vi "Serialize - Text.vi"(8 "error in (no error)":errorcluster, 11 "CRDS Data in":refnum<class "CRDS Data.lvclass">) -> (0 "error out":errorcluster, 2 "Serialized Text":string, 3 "CRDS Data out":refnum<class "CRDS Data.lvclass">)   [LabVIEW 2014, in "CRDS Lib.lvlib" / "CRDS Data.lvclass"]
uses:
  CRDS Data.lvclass
  CRDS Data.lvclass/CRDS Data.ctl
  Cell/CRDS Cell Data.lvclass
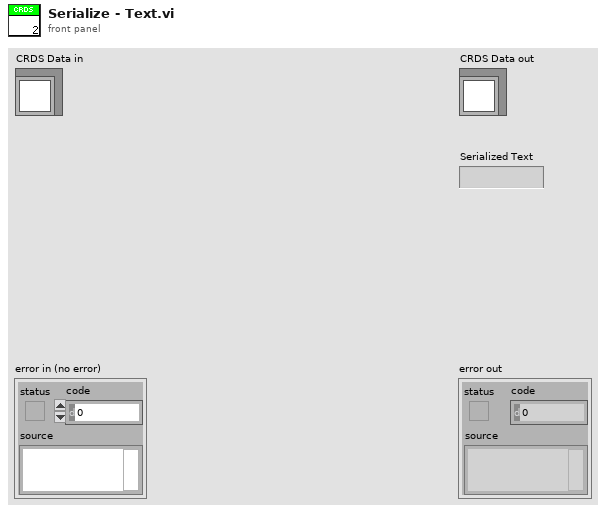
[diagram p1: front panel]
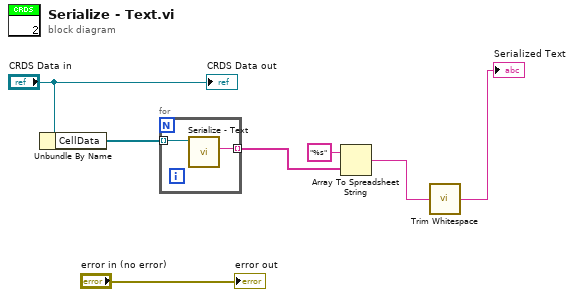
[diagram p0: block diagram]
diagram:
  n1 = Unbundle By Name("CRDS Data in") -> ("CellData"=w5:refnum<class "CRDS Cell Data.lvclass">[])
  n2 = for {
    tunnel: w5 -> [w9] mode=indexing
    tunnel: [w8] -> w4 mode=indexing
    n3 = call-dynamic "Serialize - Text.vi"("CRDS Cell Data in"=w9) -> ("Serialized Text"=w8:string)  [unwired: 8 in, 2 out]
  }
  n4 = Array To Spreadsheet String(array=w4, 3:"%s" ("format string")) -> (spreadsheet string=w2:string)  [unwired: 1 in]
  n5 = call <vilib>:"Trim Whitespace.vi"("string"=w2) -> ("trimmed string"=→"Serialized Text":string)  [unwired: 1 in]
  "error out" <- "error in (no error)"
  "CRDS Data out" <- "CRDS Data in"
